vi "Launch Subordinate.vi"(6 "Position":T1, 8 "error in":errorcluster, 9 "Panel Definiton":T3, 10 "Identifier":string, 11 "Base Software in":refnum<class "Main.lvclass">) -> (0 "error out":errorcluster, 2 "Subordinate":T2, 3 "Base Software out":refnum<class "Main.lvclass">)   [LabVIEW 2023, in "Main.lvlib" / "Main.lvclass"]
uses:
  Project/Main.lvclass
  builds/Engine/Panel Manager.lvlibp/Panel Actor/Panel Actor.lvclass
  C:/Users/Public/Documents/Development/builds/Engine/Actor Framework.lvlibp/1abvi3w/vi.lib/ActorFramework/Actor/Actor.lvclass
  builds/Engine/Panel.lvlibp/Panel/Panel.lvclass
  Custom Controls/Subordinate.ctl
  builds/Engine/Actor Framework.lvlibp/1abvi3w/vi.lib/ActorFramework/Message Enqueuer/Message Enqueuer.lvclass
  Custom Controls/Panel_Positions.ctl
  builds/Engine/Actor Framework.lvlibp/1abvi3w/vi.lib/ActorFramework/Actor/Write Actor Label.vi
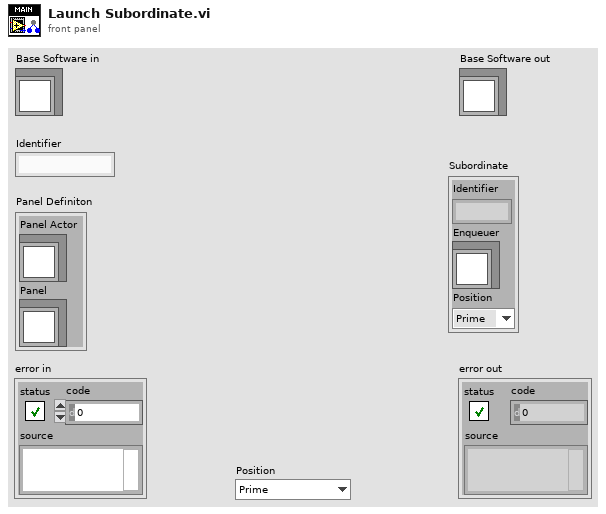
[diagram p1: front panel]
types:
  T1 = typedef "Main.lvlib/Main.lvclass/Panel_Positions.ctl" = enum16{"Prime", "Right", "Bottom", "Left", "Mission"}
  T2 = typedef "Main.lvlib/Main.lvclass/Subordinate.ctl" = cluster{"Identifier":string, "Enqueuer":refnum<class "Message Enqueuer.lvclass">, "Position":T1}
  T3 = cluster{"Panel Actor":refnum<class "Panel Actor.lvclass">, "Panel":refnum<class "Panel.lvclass">}
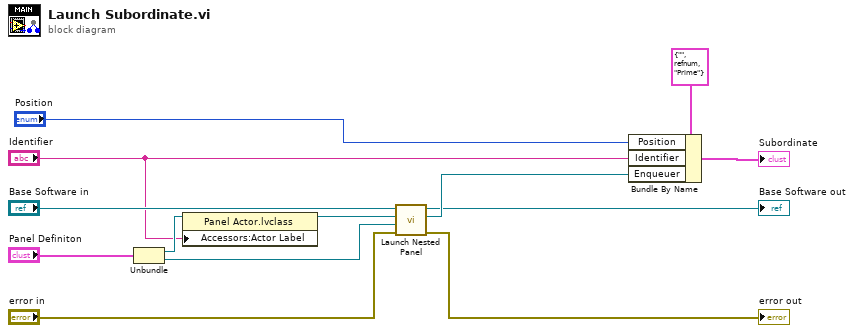
[diagram p0: block diagram]
diagram:
  n1 = Unbundle("Panel Definiton") -> ("Panel Actor"=w7:refnum<class "Panel Actor.lvclass">, "Panel"=w4:refnum<class "Panel.lvclass">)
  n2 = property class="Panel Actor.lvclass"(reference=w7, "Accessors:Actor Label"="Identifier") -> (reference out=w6:refnum<class "Panel Actor.lvclass">)  [unwired: 1 in, 1 out]
  n3 = call "Launch Nested Panel.vi"("error in (no error)"="error in", "Panel"=w4, "Nested Panel Actor"=w6, "Panel Actor in"="Base Software in") -> ("error out"=→"error out":errorcluster, "Nested Actor's Enqueuer"=w12:refnum<class "Message Enqueuer.lvclass">, "Panel Actor out"=→"Base Software out":refnum<class "Main.lvclass">)  [unwired: 4 in, 1 out]
  n4 = Bundle By Name(cluster=T2 {"Identifier"="", "Enqueuer"=refnum, "Position"=enum."Prime"} ("Subordinate"), "Position"="Position", "Identifier"="Identifier", "Enqueuer"=w12) -> (→"Subordinate":T2)
